vi "Begin.vi"(8 "error in":errorcluster) -> (0 "error out":errorcluster)   [LabVIEW 2015]
doc: "Called before other user functions, this VI is expected to open initial I/O refnums, load in file data, and do all program initialization. Notice that the <B>error out</B> terminal is simply used for data flow. Wiring it to other structures or subVIs ensures that this VI runs first."
uses:
  <vilib>/Rock Robotics/WPI/DriverStation/WPI_DriverStationRobotMode2.ctl
  <vilib>/Rock Robotics/WPI/Joystick/WPI_JoystickDeviceEnum.ctl
  <vilib>/Rock Robotics/SystemInterfaces/DIO/FPGA_DIOChannel.ctl
  <vilib>/Rock Robotics/SystemInterfaces/AI/FPGA_AIGyroChannel.ctl
  <vilib>/Rock Robotics/WPI/Solenoid/WPI_SolenoidChannel.ctl
  <vilib>/Rock Robotics/SystemInterfaces/AI/FPGA_AIChannel.ctl
  Robot Global Data.vi
  <vilib>/Rock Robotics/Network Tables/NT Write String Array.vi
  <vilib>/Rock Robotics/WPI/Counter/WPI_CounterDigitalInputToDigitalSource.vi
  <vilib>/Rock Robotics/WPI/Gyro/WPI_GyroAnalogOpen.vi
  <vilib>/Rock Robotics/WPI/Solenoid/WPI_SolenoidOpenSingle.vi
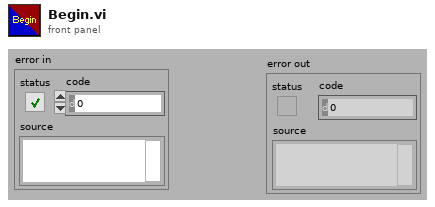
[diagram p1: front panel]
types:
  T1 = typedef "FPGA_DIOChannel.ctl" = enum8{"DIO 0", "DIO 1", "DIO 2", "DIO 3", "DIO 4", "DIO 5", "DIO 6", "DIO 7", "DIO 8", "DIO 9", "DIO MXP 0", "DIO MXP 1", "DIO MXP 2", "DIO MXP 3", "DIO MXP 4", "DIO MXP 5", "DIO MXP 6", "DIO MXP 7", "DIO MXP 8", "DIO MXP 9", "DIO MXP 10", "DIO MXP 11", "DIO MXP 12", "DIO MXP 13", "DIO MXP 14", "DIO MXP 15", "Invalid"}
  T2 = typedef "WPI_SolenoidChannel.ctl" = enum8{"Solenoid 0", "Solenoid 1", "Solenoid 2", "Solenoid 3", "Solenoid 4", "Solenoid 5", "Solenoid 6", "Solenoid 7", "Invalid"}
  T3 = cluster{"PushSolenoid":T2, "AngleMotor":cluster{"AngleMotor#":u8, "Invert AngleMotor?":bool, "PotScale":u32}, "Wheels":cluster{"LeftWheel#":u8, "Invert LeftWheel?":bool, "RightWheel#":u8, "Invert RightWheel?":bool, "WheelEncoderScale":u32}, "AnglePID":cluster{dbl, dbl, dbl}, "WheelPID":cluster{dbl, dbl, dbl}, "TopHallDIO":T1, "BottomHallDIO":T1}
  T4 = cluster{"AngleMotor#":u8, "Invert AngleMotor?":bool, "PotScale":u32}
  T5 = cluster{"LeftWheel#":u8, "Invert LeftWheel?":bool, "RightWheel#":u8, "Invert RightWheel?":bool, "WheelEncoderScale":u32}
  T6 = typedef "FPGA_AIChannel.ctl" = enum8{"AI 0", "AI 1", "AI 2", "AI 3", "AI MXP 0", "AI MXP 1", "AI MXP 2", "AI MXP 3", "Invalid"}
  T7 = cluster{"Front Right Motor Inverted":bool, "Front Left Motor Inverted":bool, "Rear Right Motor Inverted":bool, "Rear Left Motor Inverted":bool, "Middle Right Motor Inverted":bool, "Middle Left Motor Inverted":bool, "Rear Left Motor":u8, "Rear Right Motor":u8, "Front Left Motor":u8, "Front Right Motor":u8, "Middle Left Motor":u8, "Middle Right Motor":u8}
  T8 = typedef "FPGA_AIGyroChannel.ctl" = enum8{"AI 0", "AI 1", "Invalid"}
  T9 = typedef "WPI_JoystickDeviceEnum.ctl" = enum16{"USB 0", "USB 1", "USB 2", "USB 3", "USB 4", "USB 5"}
  T10 = typedef "WPI_DriverStationRobotMode2.ctl" = enum16{"Autonomous Disabled", "Autonomous Enabled", "Teleop Disabled", "Teleop Enabled", "Disconnected", "Finish", "Test Disabled", "Test Enabled", "Emergency Stopped"}
  T11 = typedef "WPI_DigitalInputDevRef.ctl" = cluster{"DevStatus":errorcluster, "DIO Channel":T1}
  T12 = typedef "FPGA_CounterEncoderSourceConvertionLVSourceType.ctl" = cluster{"DevStatus":errorcluster, "AnalogTriggerMode?":bool, "DigitalMode":cluster{"DIO Channel":T13}, "AnalogTriggerMode":cluster{"AnalogTriggerIndex":T14, "OutputType":T15}}
  T13 = typedef "FPGA_DIODigitalSourceChannel.ctl" = enum8{"DIO 0", "DIO 1", "DIO 2", "DIO 3", "DIO 4", "DIO 5", "DIO 6", "DIO 7", "DIO 8", "DIO 9", "DIO MXP 0", "DIO MXP 1", "DIO MXP 2", "DIO MXP 3", "DIO MXP 4", "DIO MXP 5", "DIO MXP 6", "DIO MXP 7", "DIO MXP 8", "DIO MXP 9", "DIO MXP 10", "DIO MXP 11", "DIO MXP 12", "DIO MXP 13", "DIO MXP 14", "DIO MXP 15", "Disabled"}
  T14 = typedef "FPGA_AnalogTriggerIndex.ctl" = enum8{"Trig 0", "Trig 1", "Trig 2", "Trig 3", "Trig 4", "Trig 5", "Trig 6", "Trig 7", "Invalid"}
  T15 = typedef "FPGA_AnalogTriggerOutType.ctl" = enum16{"InWindow", "TriggerState", "Rising", "Falling"}
  T16 = typedef "WPI_GyroDevRef.ctl" = cluster{"DevStatus":errorcluster, "Analog Channel":T6, "Offset":dbl, "Gain (VoltsPerDegree/Second)":dbl, "Gyro Type":enum16{"Analog", "XRS450"}, "Handle":i32, "SPI Bus":T17, "Device Found":bool, "Sample Rate":dbl, "Calibrate On Open":bool}
  T17 = typedef "spi_bus.ctl" = enum16{"SPI On-Board, CS0", "SPI On-Board, CS1", "SPI On-Board, CS2", "SPI On-Board, CS3", "SPI MXP", "Invalid"}
  T18 = typedef "WPI_SolenoidDevRef.ctl" = cluster{"DevStatus":errorcluster, "Pneumatics Control Module":u8, "Forward Solenoid Channel":T2, "Reverse Solenoid Channel":T2}
  T19 = typedef "WPI_EncoderDevRef.ctl" = cluster{"DevStatus":errorcluster, "EncoderIndex":T20, "CounterIndex":T21, "DistancePerCount":dbl, "Decoding Type":T22}
  T20 = typedef "FPGA_EncoderIdx.ctl" = enum8{"Enc 0", "Enc 1", "Enc 2", "Enc 3", "Enc 4", "Enc 5", "Enc 6", "Enc 7", "Invalid"}
  T21 = typedef "FPGA_CounterCtrSystemIndex.ctl" = enum8{"Ctr 0", "Ctr 1", "Ctr 2", "Ctr 3", "Ctr 4", "Ctr 5", "Ctr 6", "Ctr 7", "Invalid"}
  T22 = typedef "WPI_EncoderType.ctl" = enum16{"1x", "2x", "4x"}
  T23 = typedef "WPI_JoystickDevRef.ctl" = cluster{"Device":T9}
  T24 = typedef "WPI_PotentiometerDevRef.ctl" = cluster{"DevStatus":errorcluster, "Analog Channel":T6, "Invert Output":bool}
  T25 = typedef "WPI_SerialPortRef.ctl" = cluster{"DevStatus":errorcluster, "Serial Port Name":refnum<visa-resource-name>}
  T26 = typedef "WPI_RobotDriveDevRef.ctl" = cluster{"DevStatus":errorcluster, "Motors[]":T27[], "Square Inputs":bool, "Max Output":dbl}
  T27 = typedef "WPI_MotorControlDeviceRef.ctl" = cluster{"DeviceStatus":errorcluster, "Type":T28, "PWM":cluster{"PWM Channel":T29, "DeadBand":T30}, "CAN":cluster{"Device Number":u8, "Control Mode":T31, "Semaphore":T32, "Max Vout":dbl, "TalonSRX Control Mode":T33}, "Invert":bool}
  T28 = typedef "WPI_MotorControlType.ctl" = enum16{"PWM", "CAN", "CANTalonSRX"}
  T29 = typedef "FPGA_DIOPWMChannel.ctl" = enum8{"PWM 0", "PWM 1", "PWM 2", "PWM 3", "PWM 4", "PWM 5", "PWM 6", "PWM 7", "PWM 8", "PWM 9", "PWM MXP 0", "PWM MXP 1", "PWM MXP 2", "PWM MXP 3", "PWM MXP 4", "PWM MXP 5", "PWM MXP 6", "PWM MXP 7", "PWM MXP 8", "PWM MXP 9", "Invalid"}
  T30 = typedef "WPI_PWMDeadband.ctl" = cluster{"Name":string, "maxPositivePwm":i32, "minPositivePwm":i32, "centerPwm":i32, "maxNegativePwm":i32, "minNegativePwm":i32, "angularRange":u16}
  T31 = typedef "WPI_CANJaguar_ControlMode.ctl" = enum8{"Percent VBus", "Current", "Speed", "Position", "Voltage"}
  T32 = typedef "Semaphore RefNum" = refnum<k1>
  T33 = typedef "WPI_CANTalonSRX_APIControlMode.ctl" = enum8{"Percent VBus", "Speed", "Position", "Slave", "Unchanged / Invalid", "Voltage Compensation", "Current", "Motion Profile"}
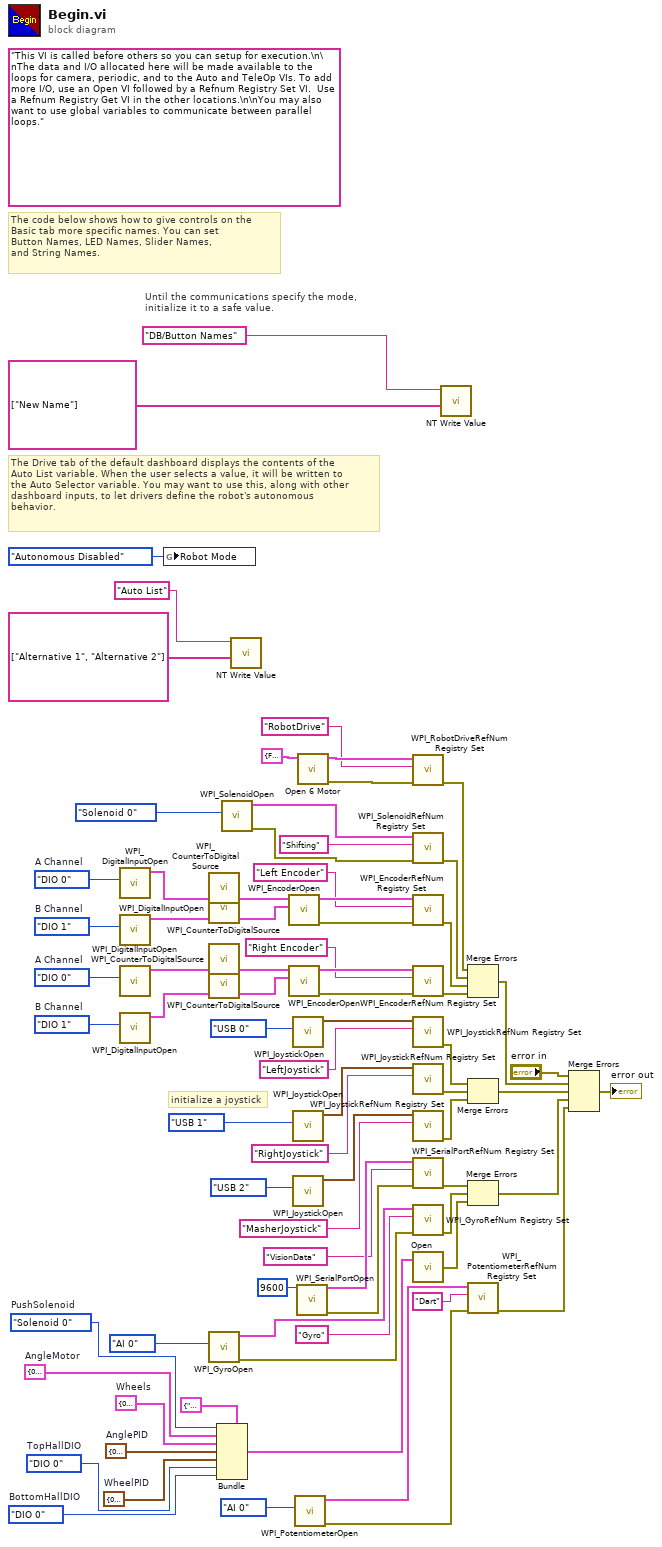
[diagram p0: block diagram]
diagram:
  w3 = FPGA_DIOChannel."DIO 0"  # BottomHallDIO
  w4 = FPGA_DIOChannel."DIO 0"  # TopHallDIO
  w7 = T4 {"AngleMotor#"=0, "Invert AngleMotor?"=FALSE, "PotScale"=0}  # AngleMotor
  w8 = T5 {"LeftWheel#"=0, "Invert LeftWheel?"=FALSE, "RightWheel#"=0, "Invert RightWheel?"=FALSE, "WheelEncoderScale"=0}  # Wheels
  w11 = WPI_SolenoidChannel."Solenoid 0"  # PushSolenoid
  w9 = cluster{dbl, dbl, dbl} {0.0, 0.0, 0.0}  # WheelPID
  w10 = cluster{dbl, dbl, dbl} {0.0, 0.0, 0.0}  # AnglePID
  w57 = FPGA_DIOChannel."DIO 1"  # B Channel
  w56 = FPGA_DIOChannel."DIO 0"  # A Channel
  w63 = FPGA_DIOChannel."DIO 1"  # B Channel
  w62 = FPGA_DIOChannel."DIO 0"  # A Channel
  (unwired) "This VI is called before others so you can setup for execution.\n\nThe data and I/O allocated here will be made available to the loops for camera, periodic, and to the Auto and TeleOp VIs. To add more I/O, use an Open VI followed by a Refnum Registry Set VI.  Use a Refnum Registry Get VI in the other locations.\n\nYou may also want to use global variables to communicate between parallel loops."
  # "The Drive tab of the default dashboard displays the contents of the\nAuto List variable. When the user selects a value, it will be written to\nthe Auto Selector variable. You may want to use this, along with other\ndashboard inputs, to let drivers define the robot's autonomous\nbehavior."
  # "The code below shows how to give controls on the\nBasic tab more specific names. You can set\nButton Names, LED Names, Slider Names,\nand String Names."
  # "initialize a joystick"
  # "Until the communications specify the mode,\ninitialize it to a safe value."
  n1 = call <vilib>:"WPI_DigitalInputOpen.vi"("DIO Channel"=w62) -> ("DigitalInputDevRef"=w59:T11)  [unwired: 1 in, 9 out]
  n2 = call <vilib>:"WPI_DigitalInputOpen.vi"("DIO Channel"=w63) -> ("DigitalInputDevRef"=w60:T11)  [unwired: 1 in, 9 out]
  n3 = call <vilib>:"WPI_DigitalInputOpen.vi"("DIO Channel"=w56) -> ("DigitalInputDevRef"=w53:T11)  [unwired: 1 in, 9 out]
  n4 = call <vilib>:"WPI_DigitalInputOpen.vi"("DIO Channel"=w57) -> ("DigitalInputDevRef"=w54:T11)  [unwired: 1 in, 9 out]
  n5 = global write "Robot Global Data.vi" "Robot Mode"(WPI_DriverStationRobotMode2."Autonomous Disabled" ("Robot Mode")) -> ()
  n6 = call-poly <vilib>:"WPI_CounterToDigitalSource.vi"("DigitalInputDevRef"=w59) -> ("Digital Source"=w58:T12)  [unwired: 6 out]
  n7 = call-poly <vilib>:"WPI_CounterToDigitalSource.vi"("DigitalInputDevRef"=w60) -> ("Digital Source"=w61:T12)  [unwired: 6 out]
  n8 = call-poly <vilib>:"WPI_CounterToDigitalSource.vi"("DigitalInputDevRef"=w53) -> ("Digital Source"=w52:T12)  [unwired: 6 out]
  n9 = call-poly <vilib>:"WPI_CounterToDigitalSource.vi"("DigitalInputDevRef"=w54) -> ("Digital Source"=w55:T12)  [unwired: 6 out]
  n10 = call-poly <vilib>:"WPI_GyroOpen.vi"("Analog Channel"=FPGA_AIGyroChannel."AI 0") -> ("error out"=w49:errorcluster, "GyroDevRef"=w51:T16)  [unwired: 8 in, 1 out]
  n11 = Bundle(cluster=T3 {"PushSolenoid"=enum."Solenoid 0", "AngleMotor"={"AngleMotor#"=0, "Invert AngleMotor?"=FALSE, "PotScale"=0}, "Wheels"={"LeftWheel#"=0, "Invert LeftWheel?"=FALSE, "RightWheel#"=0, "Invert RightWheel?"=FALSE, "WheelEncoderScale"=0}, "AnglePID"={0.0, 0.0, 0.0}, "WheelPID"={0.0, 0.0, 0.0}, "TopHallDIO"=enum."DIO 9", "BottomHallDIO"=enum."DIO 8"} ("input cluster"), "PushSolenoid"=w11, "AngleMotor"=w7, "Wheels"=w8, "AnglePID"=w10, "WheelPID"=w9, "TopHallDIO"=w4, "BottomHallDIO"=w3) -> (w2:T3)
  n12 = call-poly <vilib>:"WPI_SolenoidOpen.vi"("Solenoid Channel"=WPI_SolenoidChannel."Solenoid 0") -> ("error out"=w43:errorcluster, "SolenoidDevRef"=w44:T18)  [unwired: 9 in]
  n13 = call-poly <vilib>:"NT Write Value.vi"("String Array"=string[] ["Alternative 1", "Alternative 2"], "Name"="Auto List") -> ()  [unwired: 9 in, 1 out]
  n14 = call <vilib>:"WPI_EncoderOpen.vi"("BSource"=w61, "ASource"=w58) -> ("error out"=w48:errorcluster, "EncoderDevRef"=w47:T19)  [unwired: 6 in, 2 out]
  n15 = call <vilib>:"WPI_EncoderOpen.vi"("BSource"=w55, "ASource"=w52) -> ("error out"=w45:errorcluster, "EncoderDevRef"=w46:T19)  [unwired: 6 in, 2 out]
  n16 = call <vilib>:"WPI_JoystickOpen.vi"("JoystickDevice"=WPI_JoystickDeviceEnum."USB 0") -> ("JoystickDevRef"=w75:T23)  [unwired: 10 in]
  n17 = call <vilib>:"WPI_JoystickOpen.vi"("JoystickDevice"=WPI_JoystickDeviceEnum."USB 1") -> ("JoystickDevRef"=w68:T23)  [unwired: 10 in]
  n18 = call <vilib>:"WPI_JoystickOpen.vi"("JoystickDevice"=WPI_JoystickDeviceEnum."USB 2") -> ("JoystickDevRef"=w65:T23)  [unwired: 10 in]
  n19 = call <vilib>:"WPI_PotentiometerOpen.vi"("Analog Channel"=FPGA_AIChannel."AI 0") -> ("error out"=w29:errorcluster, "PotDevRef"=w28:T24)  [unwired: 9 in]
  n20 = call <vilib>:"WPI_SerialPortOpen.vi"("Baud Rate"=u32 9600) -> ("SerialPortRef"=w35:T25, "error out"=w36:errorcluster)  [unwired: 13 in]
  n21 = call "Open 6 Motor.vi"("Cluster"=T7 {"Front Right Motor Inverted"=FALSE, "Front Left Motor Inverted"=FALSE, "Rear Right Motor Inverted"=FALSE, "Rear Left Motor Inverted"=FALSE, "Middle Right Motor Inverted"=FALSE, "Middle Left Motor Inverted"=FALSE, "Rear Left Motor"=0, "Rear Right Motor"=0, "Front Left Motor"=0, "Front Right Motor"=0, "Middle Left Motor"=0, "Middle Right Motor"=0}) -> ("error out"=w30:errorcluster, "RobotDriveDevRef"=w32:T26)  [unwired: 9 in]
  n22 = call <vilib>:"WPI_RobotDriveRefNum Registry Set.vi"("error in (no error)"=w30, "refnum name"="RobotDrive", "RobotDriveDevRef"=w32) -> ("error out"=w22:errorcluster)  [unwired: 7 in, 1 out]
  n23 = call <vilib>:"WPI_SolenoidRefNum Registry Set.vi"("error in (no error)"=w43, "refnum name"="Shifting", "SolenoidDevRef"=w44) -> ("error out"=w21:errorcluster)  [unwired: 7 in, 1 out]
  n24 = call <vilib>:"WPI_EncoderRefNum Registry Set.vi"("error in (no error)"=w48, "refnum name"="Left Encoder", "EncoderDevRef"=w47) -> ("error out"=w20:errorcluster)  [unwired: 7 in, 1 out]
  n25 = call <vilib>:"WPI_EncoderRefNum Registry Set.vi"("error in (no error)"=w45, "refnum name"="Right Encoder", "EncoderDevRef"=w46) -> ("error out"=w19:errorcluster)  [unwired: 7 in, 1 out]
  n26 = call <vilib>:"WPI_JoystickRefNum Registry Set.vi"("refnum name"="LeftJoystick", "JoystickDevRef"=w75) -> ("error out"=w25:errorcluster)  [unwired: 8 in, 1 out]
  n27 = call <vilib>:"WPI_JoystickRefNum Registry Set.vi"("refnum name"="RightJoystick", "JoystickDevRef"=w68) -> ("error out"=w24:errorcluster)  [unwired: 8 in, 1 out]
  n28 = call <vilib>:"WPI_JoystickRefNum Registry Set.vi"("refnum name"="MasherJoystick", "JoystickDevRef"=w65) -> ("error out"=w23:errorcluster)  [unwired: 8 in, 1 out]
  n29 = call <vilib>:"WPI_SerialPortRefNum Registry Set.vi"("error in (no error)"=w36, "refnum name"="VisionData", "SerialPortRef"=w35) -> ("error out"=w15:errorcluster)  [unwired: 7 in, 1 out]
  n30 = call <vilib>:"WPI_GyroRefNum Registry Set.vi"("error in (no error)"=w49, "refnum name"="Gyro", "GyroDevRef"=w51) -> ("error out"=w14:errorcluster)  [unwired: 7 in, 1 out]
  n31 = call "Open.vi"("input cluster"=w2) -> ("error out"=w13:errorcluster)  [unwired: 1 in]
  n32 = call-poly <vilib>:"NT Write Value.vi"("String Array"=string[] ["New Name"], "Name"="DB/Button Names") -> ()  [unwired: 9 in, 1 out]
  n33 = Merge Errors(w22, w21, w20, w19) -> (w16:errorcluster)
  n34 = Merge Errors(w25, w24, w23) -> (w18:errorcluster)
  n35 = Merge Errors(w15, w14, w13) -> (w12:errorcluster)
  n36 = call <vilib>:"WPI_PotentiometerRefNum Registry Set.vi"("error in (no error)"=w29, "refnum name"="Dart", "PotDevRef"=w28) -> ("error out"=w6:errorcluster)  [unwired: 7 in, 1 out]
  n37 = Merge Errors("error in", w16, w18, w12, w6) -> (→"error out":errorcluster)
